vi "DAQ Viewer-Core_Initialize.vi"(0 "Initialization Sequence":string, 5 "FTW Actor Instance Configuration":string, 11 "error in (no error)":errorcluster) -> (4 "Actor Template-Core out":refnum<class "DAQ Viewer-Core.lvclass">, 6 "Incoming Requests":refnum<event-registration>, 8 "Local Messages":refnum<event-registration>, 15 "error out":errorcluster)   [LabVIEW 2013, in "DAQ Viewer-Core.lvclass"]
uses:
  DAQ Viewer-Core.lvclass
  source/actor/Message/Request/FTW-Message-IncomingRequest.lvclass
  source/actor/Message/Base/FTW-Message.lvclass
  source/Reflection/FTW-Reflection-Type.vi
  source/JSON/FTW-JSON-Core-LibraryFilepath.vi
  source/JSON/FTW-JSON-Core-GetFlattenedValue.vi
  source/JSON/FTW-JSON-Core-LibraryError.vi
  source/CodeGen/JSON Deserialize/FTW-JSON-Deserialize.xnode
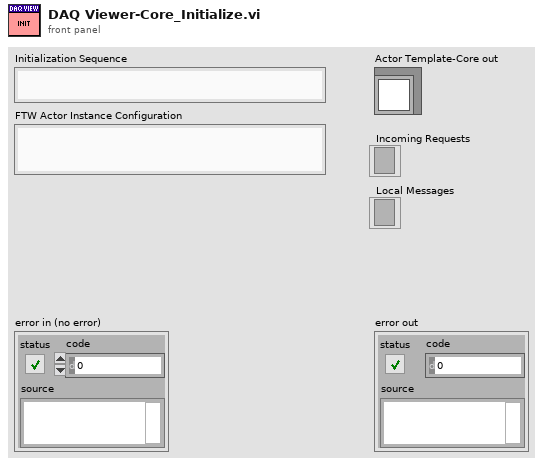
[diagram p1: front panel]
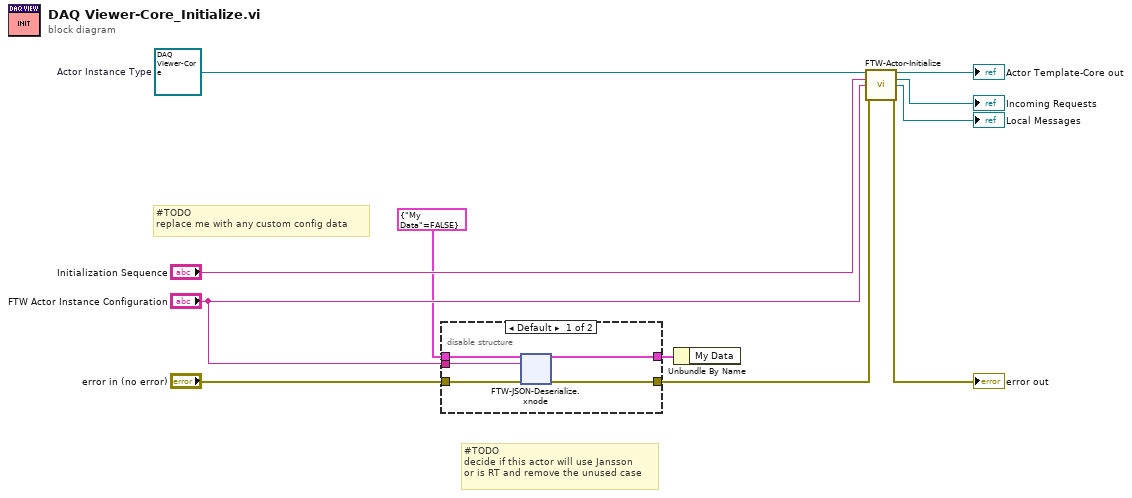
[diagram p0: block diagram]
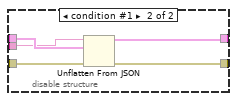
[diagram p2: hidden frame]
diagram:
  w1 = refnum<class "DAQ Viewer-Core.lvclass"> refnum  # Actor Instance Type
  # "#TODO\ndecide if this actor will use Jansson\nor is RT and remove the unused case"
  # "#TODO\nreplace me with any custom config data"
  n1 = disable-structure shown="Default" {
    disable-tunnel: "error in (no error)" -> [w16 w55]
    disable-tunnel: [w15 w54] -> w6
    disable-tunnel: "FTW Actor Instance Configuration" -> [w14 w52]
    disable-tunnel: cluster{"My Data":bool} {"My Data"=FALSE} ("Type and Defaults") -> [w13 w53]
    disable-tunnel: [w12 w51] -> w3
    frame condition #0 (active) {
      n2 = xnode "FTW-JSON-Deserialize.xnode"("Type and Defaults"=w13, "JSON String"=w14, "error in"=w16) -> ("Values"=w12:cluster{"My Data":bool}, "error out"=w15:errorcluster)
    }
    frame condition #1 {
      n3 = Unflatten From JSON(JSON string=w52, type and defaults=w53, error in (no error)=w55) -> (value=w51:cluster{"My Data":bool}, error out=w54:errorcluster)  [unwired: 4 in]
    }
  }
  n4 = Unbundle By Name(w3) -> ()  [unwired: 1 out]
  n5 = call-dynamic "FTW-Actor-Initialize.vi"("FTW Actor Instance Type"=w1, "Initialization Job Sequence"="Initialization Sequence", "Actor Instance Configuration"="FTW Actor Instance Configuration", "error in"=w6) -> ("FTW Actor Instance"=→"Actor Template-Core out":refnum<class "DAQ Viewer-Core.lvclass">, "Incoming Requests"=→"Incoming Requests":refnum<event-registration>, "Local Messages"=→"Local Messages":refnum<event-registration>, "error out"=→"error out":errorcluster)  [unwired: 8 in]
